vi "Module Init.vi"(8 "error in (no error)":errorcluster, 11 "ValveControlModule in":refnum<class "DigitalControlModule.lvclass">) -> (0 "error out":errorcluster, 3 "ValveControlModule out":refnum<class "DigitalControlModule.lvclass">)   [LabVIEW 2023, in "VolatusControl.lvlib" / "DigitalControlModule.lvclass"]
uses:
  DigitalControlModule.lvclass
  lv-vecto/Vecto/Group DBL/Group DBL.lvclass
  VolatusConfig/Meta Type.ctl
  Volatus/Module/Module.lvclass/Module.ctl
  DigitalControlModule.lvclass/DigitalControlModule.ctl
  VolatusConfig/VolatusConfigElement/VolatusConfigElement.lvclass/VolatusConfigElement.ctl
  lv-vecto/Vecto/Group/Group.lvclass/Group.ctl
  lv-vecto/Vecto/Group Config/Group Config.lvclass/Group Config.ctl
  Volatus/Module/Config.vi
  VolatusConfig/VolatusConfigElement/Element.vi
  lv-vecto/Vecto/Group Config/Get Channels.vi
  VolatusConfig/Task/Task Config.lvclass
  lv-cdm/CDM-Config/Config Lookup/Match Meta.vi
  lv-cdm/CDM-Config/Config Element/Owner.vi
  lv-cdm/CDM-Config/Config Manager/Lookup Descendant.vi
  lv-cdm/CDM-Config/Config Filter/Config Lookup.lvclass
  Volatus/MessageQ/MessageQ.lvclass
  lv-cdm/CDM-Config/Config Element/Config Element.lvclass
  Volatus/Module/Module.lvclass
  VolatusConfig/Group/Group Config.lvclass
  VolatusData/Data Processor Module/Data Processor Module.lvclass
  C:/dev/volatus/mts-volatus-super/libs/lv-volatus/Volatus/Module/Module.lvclass
  C:/dev/volatus/mts-volatus-super/libs/lv-volatus/VolatusControl/DigitalControlModule/DigitalControlModule.lvclass
  VolatusConfig/VolatusConfigElement/VolatusConfigElement.lvclass
  VolatusConfig/VolatusConfig.lvlib
  VolatusData/Data Buffer DBL/Data Buffer DBL.lvclass
  C:/dev/volatus/mts-volatus-super/libs/lv-vecto/Vecto/Group/Group.lvclass
  C:/dev/volatus/mts-volatus-super/libs/lv-vecto/Vecto/Group DBL/Group DBL.lvclass
  lv-vecto/Vecto/Group/Group.lvclass
  C:/dev/volatus/mts-volatus-super/libs/lv-volatus/VolatusConfig/VolatusConfigElement/VolatusConfigElement.lvclass
  C:/dev/volatus/mts-volatus-super/libs/lv-volatus/VolatusConfig/Task/Task Config.lvclass
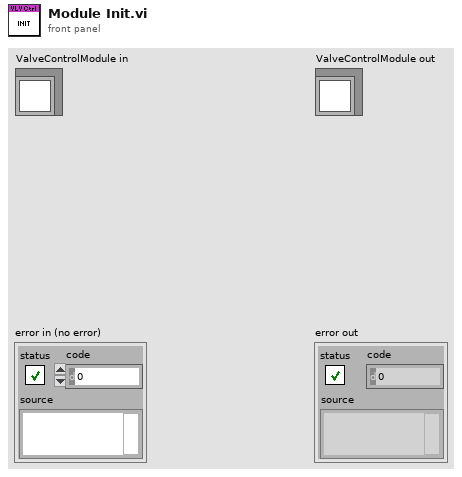
[diagram p1: front panel]
types:
  T1 = typedef "VolatusConfig.lvlib/Meta Type.ctl" = enum16{"UNKNOWN", "VL_System", "VL_Cluster", "VL_Node", "VL_Task", "VL_Group", "VL_Channel", "VL_Task_List", "VL_Scaling", "VL_Sensor", "VL_Sensor_List", "VL_Scale"}
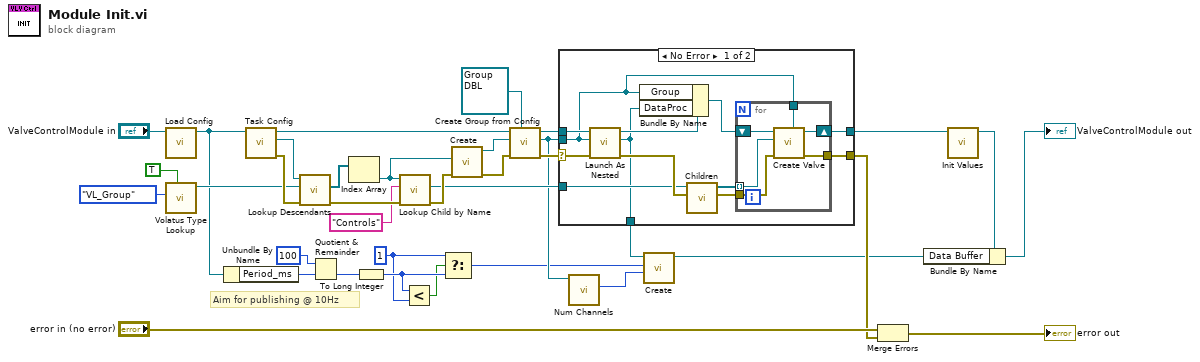
[diagram p0: block diagram]
diagram:
  w3 = 1
  # "Aim for publishing @ 10Hz"
  n1 = call "Load Config.vi"("ValveControlModule in"="ValveControlModule in") -> ("ValveControlModule out"=w14:refnum<class "DigitalControlModule.lvclass">)  [unwired: 9 in, 1 out]
  n2 = call "Volatus Type Lookup.vi"("Don't Recurse Past Match (F)"=TRUE, "Meta Type"=Meta_Type."VL_Group") -> ("Config Lookup out"=w20:refnum<class "Config Lookup.lvclass">)  [unwired: 8 in, 1 out]
  n3 = Unbundle By Name(w14) -> ("Period_ms"=w12:i64)
  n4 = call "Task Config.vi"("Module in"=w14) -> ("error out"=w36:errorcluster, "Task Config"=w29:refnum<class "Task Config.lvclass">, "Module out"=w27:refnum<class "DigitalControlModule.lvclass">)  [unwired: 8 in]
  n5 = call "Lookup Descendants.vi"("error in (no error)"=w36, "Lookup"=w20, "VolatusConfigElement in"=w29) -> ("error out"=w34:errorcluster, "Descendants"=w28:refnum<class "Config Element.lvclass">[])  [unwired: 6 in, 1 out]
  n6 = Quotient & Remainder(x=i64 100, y=w12) -> (floor(x/y)=w11:i64)  [unwired: 1 out]
  n7 = Index Array(array=w28) -> (element=w17:refnum<class "Config Element.lvclass">)  [unwired: 1 in]
  n8 = To Long Integer(number=w11) -> (32bit integer=w4:i32)
  n9 = call "Lookup Child by Name.vi"("error in (no error)"=w34, "Name"="Controls", "Config Element in"=w17) -> ("error out"=w35:errorcluster, "Child"=w15:refnum<class "Config Element.lvclass">)  [unwired: 5 in, 2 out]
  n10 = Less?(x=w4, y=w3) -> (x < y?=w2:bool)
  n11 = Select(t=w3, s=w2, f=w4) -> (s? t:f=w1:i32)
  n12 = call "Create.vi"("error in (no error)"=w35, "Element"=w17) -> ("error out"=w25:errorcluster, "Group out"=w26:refnum<class "Group Config.lvclass">)  [unwired: 8 in]
  n13 = call "Create Group from Config.vi"("Group Type (Abstract)"=refnum<class "Group DBL.lvclass"> refnum ("Vecto.lvlib:Group.lvclass"), "error in (no error)"=w25, "Group Config"=w26, "Module in"=w27) -> ("error out"=w21:errorcluster, "Group"=w9:refnum<class "Group DBL.lvclass">, "Module out"=w22:refnum<class "DigitalControlModule.lvclass">)  [unwired: 5 in]
  n14 = case shown="No Error" w21 {
    selector: w21 -> [w39 w55]
    tunnel: [w45 w55] -> w30
    tunnel: w15 -> [w44 _]
    tunnel: [w43 w56] -> w23
    tunnel: w9 -> [w38 _]
    tunnel: w22 -> [w42 w56]
    tunnel: [w37 _] -> w10
    frame No Error {
      n15 = call "Launch As Nested.vi"("error in (no error)"=w39, "Group"=w38, "Parent in"=w42) -> ("error out"=w48:errorcluster, "MessageQ"=w37:refnum<class "MessageQ.lvclass">, "Parent out"=w41:refnum<class "DigitalControlModule.lvclass">)  [unwired: 6 in]
      n16 = Bundle By Name(cluster=w41, "Group"=w38, "DataProc"=w37) -> (w40:refnum<class "DigitalControlModule.lvclass">)
      n17 = call "Children.vi"("error in (no error)"=w48, "Config Element in"=w44) -> ("error out"=w46:errorcluster, "Elements"=w47:refnum<class "Config Element.lvclass">[])  [unwired: 8 in]
      n18 = for {
        tunnel: w47 -> [w53] mode=indexing
        shift-right: [w52] -> w43
        shift-left: w40 -> [w54]
        tunnel: w46 -> [w51]
        tunnel: [w50] -> w45
        tunnel: w38 -> [w49]
        n19 = call "Create Valve.vi"("Group"=w49, "error in (no error)"=w51, "Config Element"=w53, "ValveControlModule in"=w54) -> ("error out"=w50:errorcluster, "ValveControlModule out"=w52:refnum<class "DigitalControlModule.lvclass">)  [unwired: 6 in]
      }
    }
    frame Error {
    }
  }
  n20 = call "Num Channels.vi"("Group in"=w9) -> ("Num Channels"=w8:i32)  [unwired: 8 in, 2 out]
  n21 = call "Create.vi"("# Chans"=w8, "Size"=w1, "MsgQ"=w10) -> ("Data Buffer out"=w7:refnum<class "Data Buffer DBL.lvclass">)  [unwired: 7 in, 1 out]
  n22 = Merge Errors("error in (no error)", w30) -> (→"error out":errorcluster)
  n23 = call "Init Values.vi"("ValveControlModule in"=w23) -> ("ValveControlModule out"=w6:refnum<class "DigitalControlModule.lvclass">)  [unwired: 9 in, 1 out]
  n24 = Bundle By Name(cluster=w6, "Data Buffer"=w7) -> (→"ValveControlModule out":refnum<class "DigitalControlModule.lvclass">)
